vi "Error handler-UI handling loop.vi"(8 "error in (no error)":errorcluster) -> (0 "No error":errorcluster)   [LabVIEW 2013]
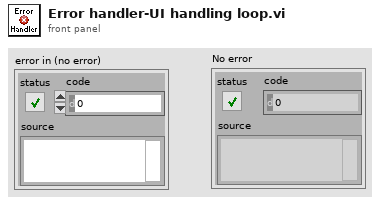
[diagram p1: front panel]
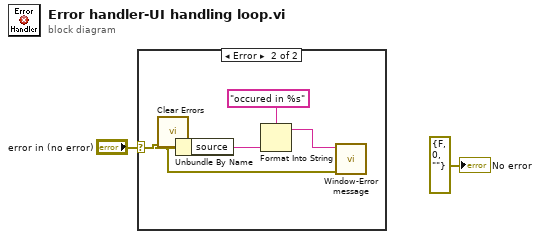
[diagram p0: block diagram]
diagram:
  n1 = case shown="Error" "error in (no error)" {
    selector: "error in (no error)" -> [_ w6]
    frame No Error {
    }
    frame Error {
      n2 = Unbundle By Name(w6) -> ("source"=w5:string)
      n3 = Format Into String(format string="occured in %s", w5) -> (resulting string=w4:string)  [unwired: 2 in, 1 out]
      n4 = call "Window-Error message.vi"("error in (no error)"=w6, "Message"=w4) -> ()  [unwired: 9 in, 1 out]
    }
  }
  n5 = call <vilib>:"Clear Errors.vi"("error in (no error)"="error in (no error)") -> ()  [unwired: 6 in, 1 out]
  "No error" <- errorcluster {"status"=FALSE, "code"=0, "source"=""} ("No error")
